vi "UpdatePSF.vi"(4 "Gaussian Profile?":bool, 5 "Edge Roll-off (dB)":dbl=10.0, 6 "Powers of 2 higher":i32=1, 7 "Window":T2=enum."Hamming", 8 "Zero-Pad the FFT?":bool, 9 "Index of Refraction":dbl=1.0 format="%_3g", 10 "Spacing (GHz)":dbl=0.1 format="%_6g", 11 "Interferometer":dbl[](array[numeric])) -> (0 "Phase Angle (rad)":dbl[](array[numeric]), 1 "X-resolution (mm)":dbl, 2 "PSF DataOut":T1, 3 "FFT":cluster{dbl[], dbl[]}(graph))   [LabVIEW 2011]
doc: "This VI analyzes an interferogram and produces the PSF and statistics about the strongest reflection in the data set.\n\nINPUTS\n1) Interferometer data\n2) Sample Pt Spacing (GHz)\n3) Index of Refraction - default is 1.0\n4) FFT control parameters\n 4.1) Apply a Gaussian Profile to the Time Record?\n 4.2) Edge Roll-off to apply to the Gaussian Profile (dB)\n 4.3) Window to apply to the Time Record (done after the Gaussian profile)\n 4.4) Zero-pad the time record?\n 4.5) What power of 2 higher to zero pad the time record length\n\n\nOUTPUTS\nPSF = 20*Log(Ampl) vs. X-position\nPhase = phase angle (wrapped) at each frequency bin / x-position, radians\nFW@3dB = Full-Width at 3-dB down\nFW@20dB = Full-Width at 20-dB down\nYpeak = Maximum amplitude in the PSF, in dB.\nXpeak = Location of the maximum amplitude, in mm.\nPTSR = Peak-To-Sidelobe Ratio\nPNFR = Peak-to-Noise-Floor Ratio\nWLRange (GHz) = calculated sweep range in GHz"
uses:
  Window_Functions.ctl
  <vilib>/measure/matone.llb/Extract Single Tone Information 1 Chan.vi
  <vilib>/Analysis/2dsp.llb/Real FFT.vi
  <vilib>/Analysis/4window.llb/Gaussian Window (DBL).vi
  <vilib>/Analysis/4window.llb/Hanning Window (DBL).vi
  <vilib>/Analysis/4window.llb/Blackman-Harris Window (DBL).vi
  <vilib>/Analysis/4window.llb/Hamming Window (DBL).vi
  <vilib>/Analysis/4window.llb/Blackman Window (DBL).vi
  <vilib>/Utility/file.llb/Write To Spreadsheet File (DBL).vi
  <vilib>/Analysis/NI_AALPro.lvlib
  <vilib>/measure/NI_MAPro.lvlib
  <vilib>/Analysis/NI_AAL_SigProc.lvlib
  <vilib>/Analysis/NI_AALBase.lvlib
panel:
  in  "Pts to skip":i32=4
  out "PNFR (dB)":dbl
  out "Noise Floor (dB)":dbl format="%0.2f"
  out "Side-Lobe Location (mm)":dbl
  out "Side-Lobe Amp (dB)":dbl
  out "Xpeak":dbl
  out "Ypeak":dbl
  out "FW@20dB":dbl
  out "FW@3dB":dbl
  in  "PSFData":path=path "I:/BTDemo/PSFData.txt"
  out "PTSR (dB)":dbl
  out "Period (pts)":dbl
  out "Amplitude":dbl
  out "Freq (1/pts)":dbl
  in  "Save Data":bool
  out "Interferometer Signal":dbl[](graph)
  # "UpdatePSF"
  # "PSF Peak Finding"
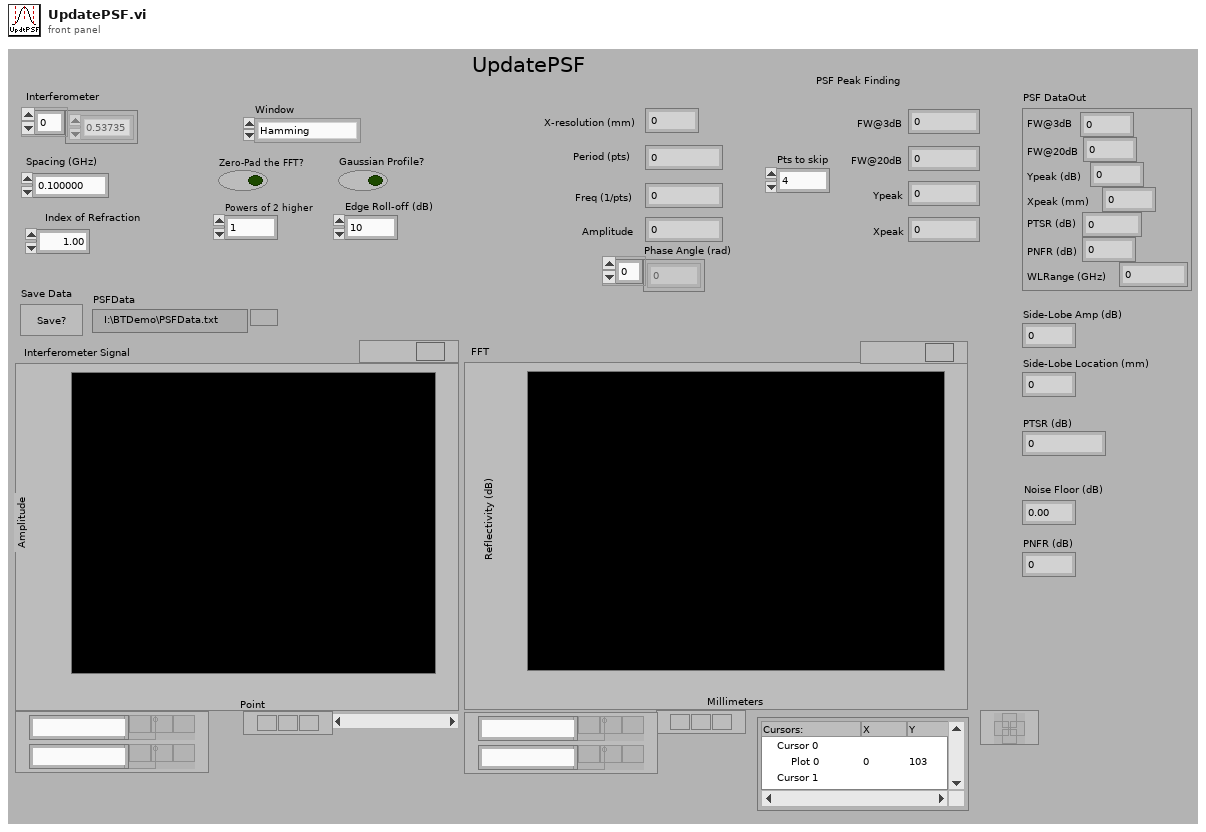
[diagram p1: front panel]
types:
  T1 = cluster{"FW@3dB":dbl, "FW@20dB":dbl, "Ypeak (dB)":dbl, "Xpeak (mm)":dbl, "PTSR (dB)":dbl, "PNFR (dB) ":dbl, "WLRange (GHz)":dbl}
  T2 = typedef "Window_Functions.ctl" = enum16{"Rectangular", "Hann", "Hamming", "Blackman", "Blackman-Harris"}
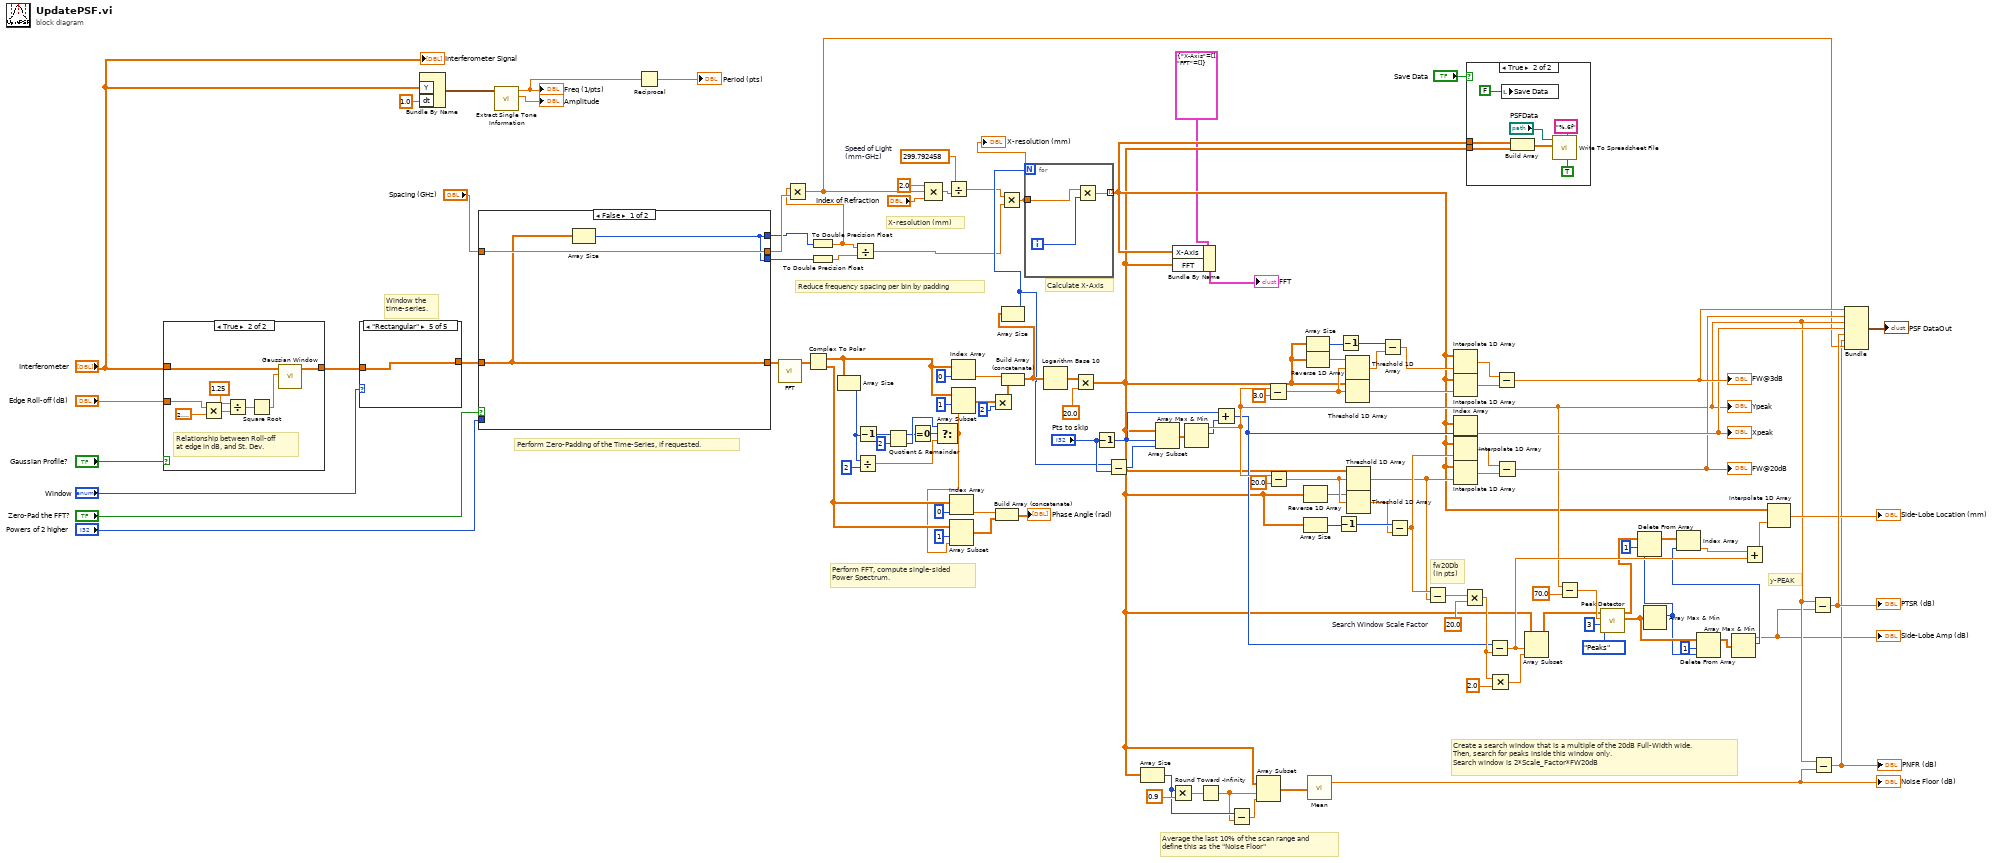
[diagram p0: block diagram]
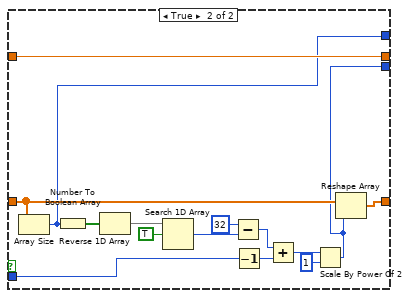
[diagram p3: hidden frame]
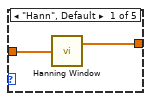
[diagram p5: hidden frame]
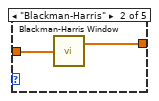
[diagram p6: hidden frame]
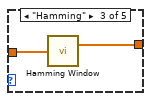
[diagram p7: hidden frame]
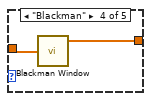
[diagram p8: hidden frame]
diagram:
  w59 = 20.0  # Search Window Scale Factor
  w72 = 299.792458  # Speed of Light  (mm-GHz)
  # "Reduce frequency spacing per bin by padding"
  # "Average the last 10% of the scan range and \ndefine this as the \"Noise Floor\""
  # "Create a search window that is a multiple of the 20dB Full-Width wide.\nThen, search for peaks inside this window only.\nSearch window is 2*Scale_Factor*FW20dB"
  # "X-resolution (mm)"
  # "fw20Db\n(in pts)"
  # "y-PEAK"
  # "Perform FFT, compute single-sided\nPower Spectrum."
  # "Window the \ntime-series."
  # "Perform Zero-Padding of the Time-Series, if requested."
  # "Calculate X-Axis"
  n1 = case shown="True" "Gaussian Profile?" {
    tunnel: [w124 w127] -> w30
    tunnel: "Interferometer" -> [w124 w126]
    tunnel: "Edge Roll-off (dB)" -> [_ w125]
    frame False {
    }
    frame True {
      # "Relationship between Roll-off \nat edge in dB, and St. Dev."
      n2 = Multiply(x=w125, y=2.302585092994046) -> (x*y=w130:dbl)
      n3 = Divide(x=1.25, y=w130) -> (x/y=w132:dbl)
      n4 = Square Root(x=w132) -> (sqrt(x)=w128:dbl)
      n5 = call-poly <vilib>:"Gaussian Window.vi"("standard deviation"=w128, "X"=w126) -> ("Windowed X"=w127:dbl[])  [unwired: 8 in, 1 out]
    }
  }
  n6 = case shown="\"Rectangular\"" "Window" {
    tunnel: [w134 w136 w137 w139 w141] -> w103
    tunnel: w30 -> [w133 w135 w138 w140 w141]
    frame "Hann", Default {
      n7 = call-poly <vilib>:"Hanning Window.vi"("X"=w133) -> ("Windowed X"=w134:dbl[])  [unwired: 1 out]
    }
    frame "Blackman-Harris" {
      n8 = call-poly <vilib>:"Blackman-Harris Window.vi"("X"=w135) -> ("Windowed X"=w136:dbl[])  [unwired: 1 out]
    }
    frame "Hamming" {
      n9 = call-poly <vilib>:"Hamming Window.vi"("X"=w138) -> ("Windowed X"=w137:dbl[])  [unwired: 1 out]
    }
    frame "Blackman" {
      n10 = call-poly <vilib>:"Blackman Window.vi"("X"=w140) -> ("Windowed X"=w139:dbl[])  [unwired: 1 out]
    }
    frame "Rectangular" {
    }
  }
  n11 = Bundle By Name("Y"="Interferometer", "dt"=1.0) -> (w116:waveform(dbl))  [unwired: 1 in]
  n12 = case shown="False" "Zero-Pad the FFT?" {
    tunnel: [w143 w159] -> w102
    tunnel: "Powers of 2 higher" -> [_ w153]
    tunnel: w103 -> [w143 w149]
    tunnel: "Spacing (GHz)" -> [w144 w147]
    tunnel: [w144 w147] -> w70
    tunnel: [w142 w146] -> w11
    tunnel: [w142 w145] -> w5
    frame False {
      n13 = Array Size(array=w143) -> (size(s)=w142:i32)
    }
    frame True {
      n14 = Array Size(array=w149) -> (size(s)=w146:i32)
      n15 = Number To Boolean Array(number=w146) -> (Boolean array=w157:bool[])
      n16 = Reverse 1D Array(array=w157) -> (reversed array=w156:bool[])
      n17 = Search 1D Array(1D array=w156, element=TRUE) -> (index of element=w155:i32)  [unwired: 1 in]
      n18 = Subtract(x=32, y=w155) -> (x-y=w152:i32)
      n19 = Decrement(x=w153) -> (x-1=w148:i32)
      n20 = Add(x=w152, y=w148) -> (x+y=w151:i32)
      n21 = Scale By Power Of 2(n=w151, x=1) -> (x*2^n=w145:i32)
      n22 = Reshape Array(w149, w145) -> (w159:dbl[])
    }
  }
  n23 = call-poly <vilib>:"Extract Single Tone Information.vi"("time signal in"=w116) -> ("detected amplitude"=→"Amplitude":dbl, "detected frequency"=w113:dbl)  [unwired: 5 in, 4 out]
  "Freq (1/pts)" <- w113
  n24 = Reciprocal(x=w113) -> (1/x=→"Period (pts)":dbl)
  n25 = call-poly <vilib>:"FFT.vi"("X"=w102) -> ("FFT {X}"=w27:cdb[])  [unwired: 9 in, 1 out]
  n26 = Complex To Polar(r * e^(i*theta)=w27) -> (r=w26:dbl[], theta=w20:dbl[])
  n27 = To Double Precision Float(number=w11) -> (double precision float=w9:dbl)
  n28 = Multiply(x=w9, y=w70) -> (x*y=w43:dbl)
  n29 = To Double Precision Float(number=w5) -> (double precision float=w10:dbl)
  n30 = Array Size(array=w26) -> (size(s)=w71:i32)
  n31 = Divide(x=w9, y=w10) -> (x/y=w6:dbl)
  n32 = Divide(x=w71, y=2) -> (x/y=w101:dbl)
  n33 = Decrement(x=w71) -> (x-1=w95:i32)
  n34 = Quotient & Remainder(x=w95, y=2) -> (x-y*floor(x/y)=w97:i32, floor(x/y)=w99:i32)
  n35 = Equal To 0?(x=w97) -> (x = 0?=w98:bool)
  n36 = Compound Arithmetic op=MULTIPLY(2.0, w43, "Index of Refraction") -> (w73:dbl)
  n37 = Select(t=w99, s=w98, f=w101) -> (s? t:f=w19:dbl)
  n38 = Divide(x=w72, y=w73) -> (x/y=w8:dbl)
  n39 = Index Array(array=w20, index=0) -> (element=w23:dbl)
  n40 = Array Subset(array=w20, index=1, length=w19) -> (w22:dbl[])
  n41 = Index Array(array=w26, index=0) -> (element=w121:dbl)
  n42 = Array Subset(array=w26, index=1, length=w19) -> (w120:dbl[])
  n43 = Multiply(x=w120, y=2) -> (x*y=w118:dbl[])
  n44 = Build Array (concatenate)(w23, w22) -> (→"Phase Angle (rad)":dbl[])
  n45 = Multiply(x=w8, y=w6) -> (x*y=w7:dbl)
  "X-resolution (mm)" <- w7
  n46 = Build Array (concatenate)(w121, w118) -> (w69:dbl[])
  n47 = Array Size(array=w69) -> (size(s)=w12:i32)
  n48 = for {
    N: w12 -> [_]
    tunnel: [w162] -> w4 mode=indexing
    tunnel: w7 -> [w160]
    i -> [w161]
    n49 = Multiply(x=w160, y=w161) -> (x*y=w162:dbl)
  }
  n50 = Logarithm Base 10(1:w69) -> (0:w112:dbl[])
  n51 = Multiply(x=w112, y=20.0) -> (x*y=w3:dbl[])
  n52 = Decrement(x="Pts to skip") -> (x-1=w15:i32)
  n53 = Subtract(x=w12, y="Pts to skip") -> (x-y=w17:i32)
  n54 = Array Size(array=w3) -> (size(s)=w46:i32)
  n55 = Array Subset(array=w3, index=w15, length=w17) -> (w18:dbl[])
  n56 = Multiply(x=w46, y=0.9) -> (x*y=w45:dbl)
  n57 = Bundle By Name(cluster=cluster{"X-Axis":dbl[], "FFT":dbl[]} {"X-Axis"=[], "FFT"=[]}, "X-Axis"=w4, "FFT"=w3) -> (→"FFT":cluster{"X-Axis":dbl[], "FFT":dbl[]})
  n58 = Array Max & Min(array=w18) -> (max value=w49:dbl, max index (indices)=w16:i32)  [unwired: 2 out]
  "Ypeak" <- w49
  n59 = Round Toward -Infinity(1:w45) -> (0:w44:dbl)
  n60 = Add(x=w15, y=w16) -> (x+y=w14:i32)
  n61 = Subtract(x=w46, y=w44) -> (x-y=w47:dbl)
  n62 = Array Subset(array=w3, index=w44, length=w47) -> (w50:dbl[])
  n63 = Subtract(x=w49, y=3.0) -> (x-y=w87:dbl)
  n64 = Subtract(x=w49, y=20.0) -> (x-y=w82:dbl)
  n65 = Reverse 1D Array(array=w3) -> (reversed array=w81:dbl[])
  n66 = Array Size(array=w3) -> (size(s)=w79:i32)
  n67 = Array Size(array=w3) -> (size(s)=w84:i32)
  n68 = Reverse 1D Array(array=w3) -> (reversed array=w88:dbl[])
  n69 = call <vilib>:"Mean.vi"("X"=w50) -> ("mean"=w48:dbl)  [unwired: 1 out]
  "Noise Floor (dB)" <- w48
  n70 = Decrement(x=w79) -> (x-1=w80:i32)
  n71 = Decrement(x=w84) -> (x-1=w83:i32)
  n72 = Threshold 1D Array(2:w87, 3:w88) -> (0:w86:dbl)  [unwired: 1 in]
  n73 = Threshold 1D Array(2:w87, 3:w3) -> (0:w64:dbl)  [unwired: 1 in]
  n74 = Threshold 1D Array(2:w82, 3:w3) -> (0:w61:dbl)  [unwired: 1 in]
  n75 = Threshold 1D Array(2:w82, 3:w81) -> (0:w78:dbl)  [unwired: 1 in]
  n76 = Subtract(x=w83, y=w86) -> (x-y=w65:dbl)
  n77 = Subtract(x=w80, y=w78) -> (x-y=w62:dbl)
  n78 = Subtract(x=w62, y=w61) -> (x-y=w60:dbl)
  n79 = Interpolate 1D Array(1:w65, 2:w4) -> (0:w85:dbl)
  n80 = Interpolate 1D Array(1:w64, 2:w4) -> (0:w92:dbl)
  n81 = Index Array(array=w4, index=w14) -> (element=w76:dbl)
  "Xpeak" <- w76
  n82 = Interpolate 1D Array(1:w62, 2:w4) -> (0:w90:dbl)
  n83 = Interpolate 1D Array(1:w61, 2:w4) -> (0:w91:dbl)
  n84 = Multiply(x=w60, y=w59) -> (x*y=w58:dbl)
  n85 = case shown="True" "Save Data" {
    tunnel: w4 -> [_ w165]
    tunnel: w3 -> [_ w164]
    frame False {
    }
    frame True {
      n86 = local write "Save Data"(FALSE) -> ()
      n87 = Build Array(w165, w164) -> (w167:dbl[][])
      n88 = call-poly <vilib>:"Write To Spreadsheet File.vi"("transpose? (no:F)"=TRUE, "format (%.3f)"="%.6f", "2D data"=w167, "file path (dialog if empty)"="PSFData") -> ()  [unwired: 4 in, 1 out]
    }
  }
  n89 = Subtract(x=w14, y=w58) -> (x-y=w54:dbl)
  n90 = Multiply(x=w58, y=2.0) -> (x*y=w56:dbl)
  n91 = Subtract(x=w85, y=w92) -> (x-y=w77:dbl)
  "FW@3dB" <- w77
  n92 = Subtract(x=w90, y=w91) -> (x-y=w75:dbl)
  "FW@20dB" <- w75
  n93 = Array Subset(array=w3, index=w54, length=w56) -> (w63:dbl[])
  n94 = Subtract(x=w49, y=70.0) -> (x-y=w66:dbl)
  n95 = call <vilib>:"Peak Detector.vi"("peaks/valleys"=enum32{"Peaks", "Valleys"}."Peaks", "width"=3, "threshold"=w66, "X"=w63) -> ("Amplitudes"=w40:dbl[], "Locations"=w34:dbl[])  [unwired: 3 in, 3 out]
  n96 = Array Max & Min(array=w40) -> (max index (indices)=w33:i32)  [unwired: 3 out]
  n97 = Delete From Array(array=w34, length=1, index=w33) -> (array with subset deleted=w37:dbl[])  [unwired: 1 out]
  n98 = Delete From Array(array=w40, length=1, index=w33) -> (array with subset deleted=w35:dbl[])  [unwired: 1 out]
  n99 = Array Max & Min(array=w35) -> (max value=w32:dbl, max index (indices)=w36:i32)  [unwired: 2 out]
  "Side-Lobe Amp (dB)" <- w32
  n100 = Index Array(array=w37, index=w36) -> (element=w55:dbl)
  n101 = Add(x=w55, y=w54) -> (x+y=w53:dbl)
  n102 = Interpolate 1D Array(1:w53, 2:w4) -> (0:→"Side-Lobe Location (mm)":dbl)
  n103 = Subtract(x=w49, y=w32) -> (x-y=w108:dbl)
  "PTSR (dB)" <- w108
  n104 = Subtract(x=w49, y=w48) -> (x-y=w42:dbl)
  "PNFR (dB)" <- w42
  n105 = Bundle(w77, w75, w49, w76, w108, w42, w43) -> (→"PSF DataOut":cluster{dbl, dbl, dbl, dbl, dbl, dbl, dbl})  [unwired: 1 in]
  "Interferometer Signal" <- "Interferometer"
